vi "FGV_DatosMotores.vi"(8 "error in (no error)":errorcluster, 10 "Val_motor_in":T2, 11 "Estado":T1) -> (0 "error out":errorcluster, 2 "Val_motor_out":T2)   [LabVIEW 2026]
uses:
  Control/Ctr_Enc_Values.ctl
  Control/Ctrl_Motores_Valores.ctl
  Control/Ctrl_Errores.ctl
  Control/Ctrl_Fgv_DatosMotores.ctl
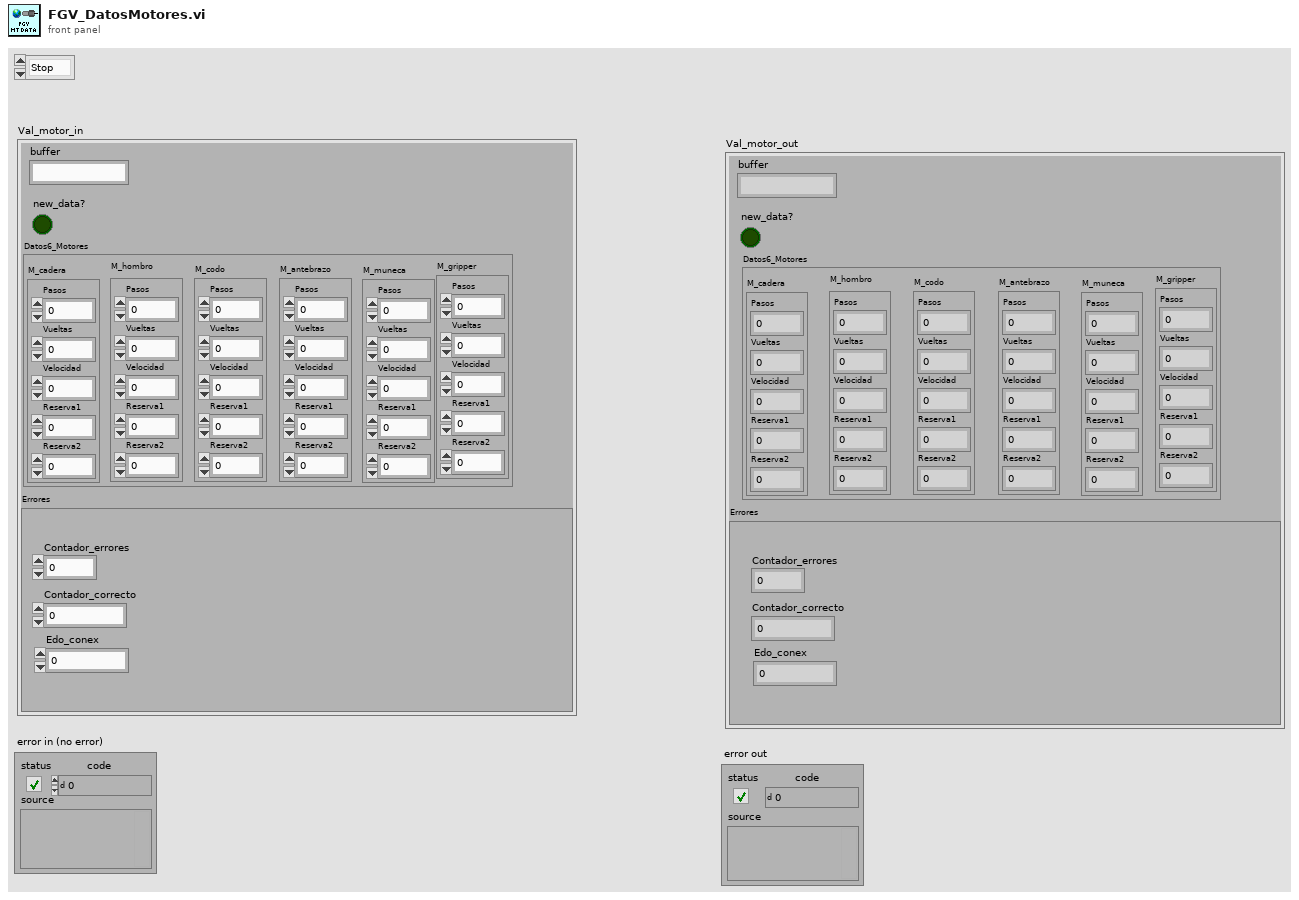
[diagram p1: front panel]
types:
  T1 = typedef "Ctrl_Fgv_DatosMotores.ctl" = enum16{"Stop", "Get", "Set"}
  T2 = typedef "Ctr_Enc_Values.ctl" = cluster{"buffer":string, "Datos6_Motores":cluster{"M_cadera":T3, "M_hombro":T3, "M_codo":T3, "M_antebrazo":T3, "M_muneca":T3, "M_gripper":T3}, "Errores":T4, "new_data?":bool}
  T3 = typedef "Ctrl_Motores_Valores.ctl" = cluster{"Pasos":i32, "Vueltas":i16, "Velocidad":i16, "Reserva1":u8, "Reserva2":u8}
  T4 = typedef "Ctrl_Errores.ctl" = cluster{"Contador_correcto":u32, "Contador_errores":u32, "Edo_conex":u32}
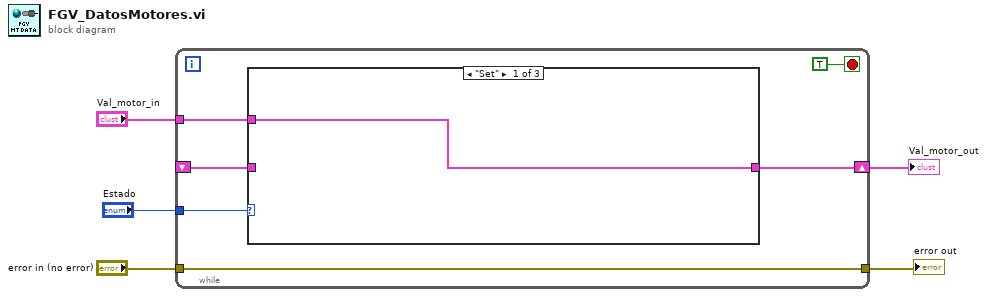
[diagram p0: block diagram]
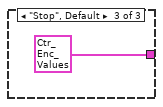
[diagram p3: hidden frame]
diagram:
  n1 = while {
    tunnel: "Estado" -> [w11]
    shift-right: [w9] -> w3
    shift-left: _ -> [w10]
    tunnel: "Val_motor_in" -> [w8]
    tunnel: "error in (no error)" -> [w6]
    tunnel: [w6] -> w1
    stop <- TRUE stop-if-true
    n2 = case shown="\"Set\"" w11 {
      tunnel: w10 -> [_ w13 _]
      tunnel: [w12 w13 T2 {"buffer"="", "Datos6_Motores"={"M_cadera"={"Pasos"=0, "Vueltas"=0, "Velocidad"=0, "Reserva1"=0, "Reserva2"=0}, "M_hombro"={"Pasos"=0, "Vueltas"=0, "Velocidad"=0, "Reserva1"=0, "Reserva2"=0}, "M_codo"={"Pasos"=0, "Vueltas"=0, "Velocidad"=0, "Reserva1"=0, "Reserva2"=0}, "M_antebrazo"={"Pasos"=0, "Vueltas"=0, "Velocidad"=0, "Reserva1"=0, "Reserva2"=0}, "M_muneca"={"Pasos"=0, "Vueltas"=0, "Velocidad"=0, "Reserva1"=0, "Reserva2"=0}, "M_gripper"={"Pasos"=0, "Vueltas"=0, "Velocidad"=0, "Reserva1"=0, "Reserva2"=0}}, "Errores"={"Contador_correcto"=0, "Contador_errores"=0, "Edo_conex"=0}, "new_data?"=FALSE} ("Val_motor_in")] -> w9
      tunnel: w8 -> [w12 _ _]
      frame "Set" {
      }
      frame "Get" {
      }
      frame "Stop", Default {
      }
    }
  }
  "Val_motor_out" <- w3
  "error out" <- w1
